vi "server_chat.vi"(1 "port":u16, 2 "queue out":refnum<queue>) -> ()   [LabVIEW 2024]
uses:
  server_state.ctl
  clients_global.vi
panel:
  in  "String":string
  in  "send":bool
  out "Numeric":i32
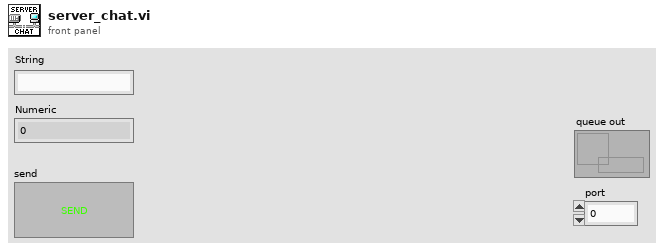
[diagram p1: front panel]
types:
  T1 = cluster{"ListenerID":refnum<k5>, "Clients":refnum<k5>[]}
  T2 = typedef "server_state.ctl" = enum16{"Init", "Connect", "Data", "Stop"}
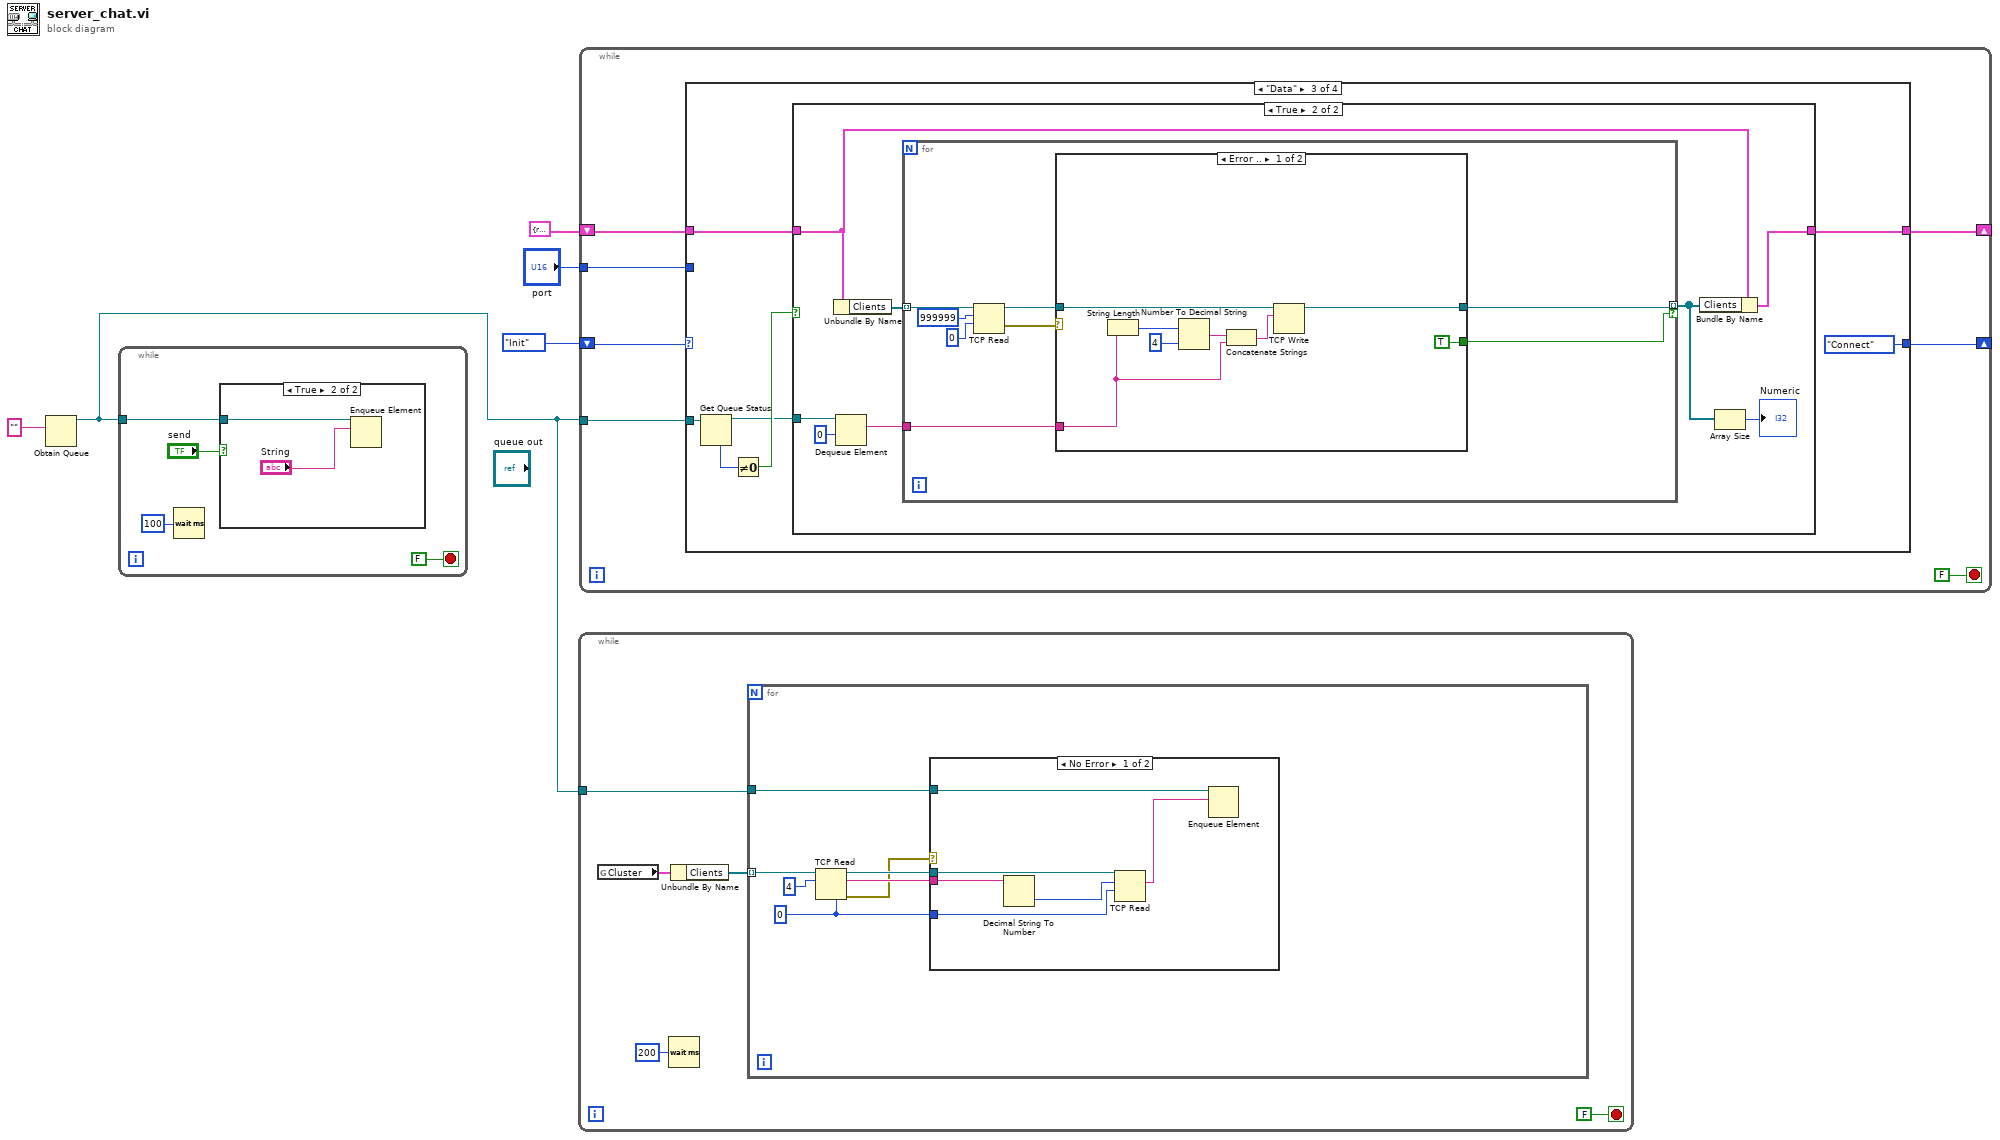
[diagram p0: block diagram]
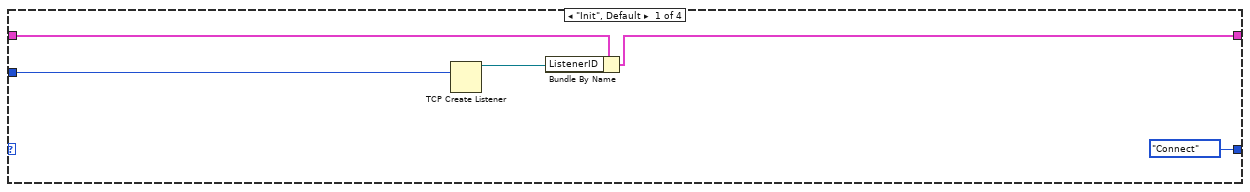
[diagram p4: hidden frame]
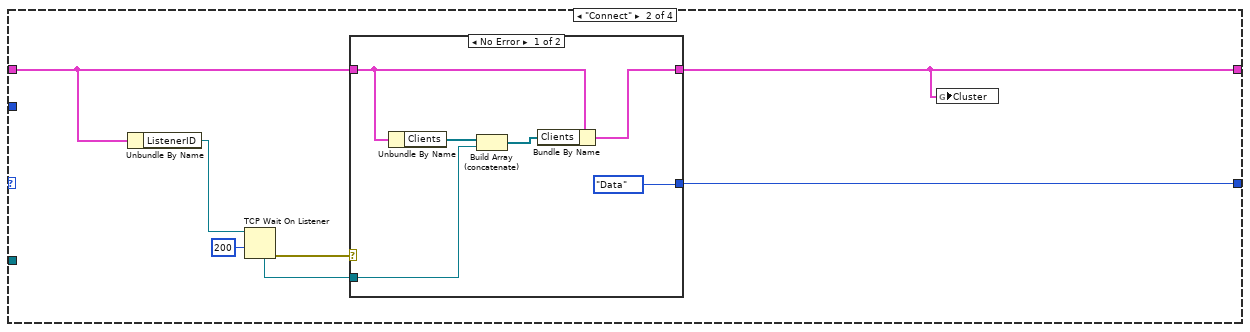
[diagram p5: hidden frame]
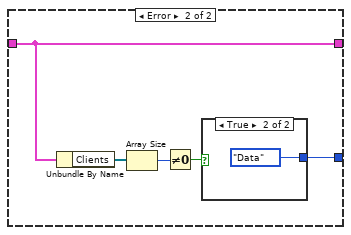
[diagram p6: hidden frame]
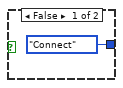
[diagram p7: hidden frame]
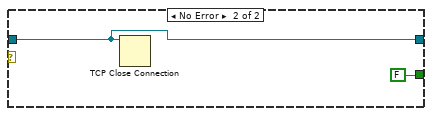
[diagram p9: hidden frame]
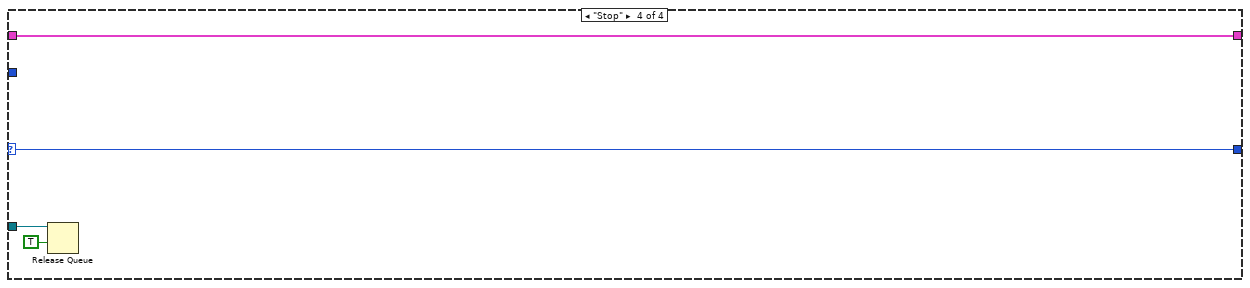
[diagram p10: hidden frame]
diagram:
  n1 = Obtain Queue(element data type="" ("name (unnamed)")) -> (queue out=w1:refnum<queue>)  [unwired: 4 in, 2 out]
  n2 = while {
    tunnel: w1 -> [w9]
    stop <- FALSE stop-if-true
    n3 = Wait (ms)(milliseconds to wait=u32 100) -> ()  [unwired: 1 out]
    n4 = case shown="True" "send" {
      tunnel: w9 -> [_ w11]
      frame False {
      }
      frame True {
        n5 = Enqueue Element(queue=w11, element="String") -> ()  [unwired: 2 in, 3 out]
      }
    }
  }
  n6 = while {
    tunnel: w1 -> [w13]
    stop <- FALSE stop-if-true
    n7 = global read "clients_global.vi" "Cluster"() -> (w14:T1)
    n8 = Wait (ms)(milliseconds to wait=u32 200) -> ()  [unwired: 1 out]
    n9 = Unbundle By Name(w14) -> ("Clients"=w15:refnum<k5>[])
    n10 = for {
      tunnel: w15 -> [w19] mode=indexing
      tunnel: w13 -> [w18]
      w23 = 0 ("timeout ms (25000)")
      n11 = TCP Read(connection ID=w19, bytes to read=4, 9:w23) -> (connection ID out=w21:refnum<k5>, data out=w20:string, error out=w17:errorcluster)  [unwired: 1 in, 1 out]
      n12 = case shown="No Error" w17 {
        tunnel: w23 -> [w29 _]
        tunnel: w21 -> [w28 _]
        tunnel: w20 -> [w27 _]
        tunnel: w18 -> [w24 _]
        frame No Error {
          n13 = Decimal String To Number(string=w27) -> (number=w26:i32)  [unwired: 2 in, 1 out]
          n14 = TCP Read(connection ID=w28, bytes to read=w26, 9:w29) -> (data out=w25:string)  [unwired: 1 in, 3 out]
          n15 = Enqueue Element(queue=w24, element=w25) -> ()  [unwired: 2 in, 3 out]
        }
        frame Error {
        }
      }
    }
  }
  n16 = while {
    shift-right: [w33] -> _
    shift-left: server_state."Init" ("Enum") -> [w36]
    shift-right: [w34] -> _
    shift-left: T1 {"ListenerID"=refnum, "Clients"=[]} -> [w35]
    tunnel: w1 -> [w31]
    tunnel: "port" -> [w30]
    stop <- FALSE stop-if-true
    n17 = case shown="\"Data\"" w36 {
      selector: w36 -> [_ _ _ w98]
      tunnel: w35 -> [w40 w46 w67 w99]
      tunnel: [w39 w42 w68 w99] -> w34
      tunnel: [server_state."Connect" ("Enum") w43 server_state."Connect" ("Enum") w98] -> w33
      tunnel: w31 -> [_ _ w65 w97]
      tunnel: w30 -> [w37 _ _ _]
      frame "Init", Default {
        n18 = TCP Create Listener(10:w37) -> (3:w38:refnum<k5>)  [unwired: 4 in, 2 out]
        n19 = Bundle By Name(cluster=w40, "ListenerID"=w38) -> (w39:T1)
      }
      frame "Connect" {
        n20 = Unbundle By Name(w46) -> ("ListenerID"=w47:refnum<k5>)
        n21 = TCP Wait On Listener(9:200 ("timeout ms (wait forever: -1)"), 11:w47) -> (0:w44:errorcluster, 4:w45:refnum<k5>)  [unwired: 2 in, 3 out]
        n22 = case shown="No Error" w44 {
          tunnel: w46 -> [w54 w59]
          tunnel: w45 -> [w51 _]
          tunnel: [w50 w59] -> w42
          tunnel: [server_state."Data" ("Enum") w55] -> w43
          frame No Error {
            n23 = Unbundle By Name(w54) -> ("Clients"=w53:refnum<k5>[])
            n24 = Build Array (concatenate)(w53, w51) -> (w52:refnum<k5>[])
            n25 = Bundle By Name(cluster=w54, "Clients"=w52) -> (w50:T1)
          }
          frame Error {
            n26 = Unbundle By Name(w59) -> ("Clients"=w58:refnum<k5>[])
            n27 = Array Size(array=w58) -> (size(s)=w57:i32)
            n28 = Not Equal To 0?(x=w57) -> (x != 0?=w56:bool)
            n29 = case shown="True" w56 {
              tunnel: [server_state."Connect" ("Enum") server_state."Data" ("Enum")] -> w55
              frame False {
              }
              frame True {
              }
            }
          }
        }
        n30 = global write "clients_global.vi" "Cluster"(w42) -> ()
      }
      frame "Data" {
        n31 = Get Queue Status(queue=w65) -> (queue out=w62:refnum<queue>, # elements in queue=w64:i32)  [unwired: 2 in, 6 out]
        n32 = Not Equal To 0?(x=w64) -> (x != 0?=w63:bool)
        n33 = case shown="True" w63 {
          tunnel: [w69 w76] -> w68
          tunnel: w67 -> [w69 w75]
          tunnel: w62 -> [_ w72]
          frame False {
          }
          frame True {
            n34 = Unbundle By Name(w75) -> ("Clients"=w77:refnum<k5>[])
            n35 = Dequeue Element(queue=w72, timeout in ms (-1)=0) -> (element=w71:string)  [unwired: 1 in, 3 out]
            n36 = for {
              tunnel: w77 -> [w85] mode=indexing
              tunnel: [w82] -> w73 mode=indexing if=w81
              tunnel: w71 -> [w78]
              n37 = TCP Read(connection ID=w85, bytes to read=999999, 9:0 ("timeout ms (25000)")) -> (connection ID out=w83:refnum<k5>, error out=w80:errorcluster)  [unwired: 2 in, 1 out]
              n38 = case shown="Error .." w80 {
                tunnel: w83 -> [w93 w95]
                tunnel: [w92 w95] -> w82
                tunnel: [TRUE FALSE] -> w81
                tunnel: w78 -> [w86 _]
                frame Error {
                  n39 = String Length(string=w86) -> (length=w90:i32)
                  n40 = Number To Decimal String(number=w90, width (-)=i16 4) -> (decimal integer string=w87:string)
                  n41 = Concatenate Strings(w87, w86) -> (w88:string)
                  n42 = TCP Write(connection ID=w93, data in=w88) -> (connection ID out=w92:refnum<k5>)  [unwired: 2 in, 2 out]
                }
                frame No Error {
                  n43 = TCP Close Connection(connection ID=w95) -> ()  [unwired: 1 in, 3 out]
                }
              }
            }
            n44 = Bundle By Name(cluster=w75, "Clients"=w73) -> (w76:T1)
            n45 = Array Size(array=w73) -> (size(s)=→"Numeric":i32)
          }
        }
      }
      frame "Stop" {
        n46 = Release Queue(queue=w97, force destroy? (F)=TRUE) -> ()  [unwired: 1 in, 3 out]
      }
    }
  }
